vi "Dashboard Main.vi"() -> ()   [LabVIEW 2019]
uses:
  <vilib>/Rock Robotics/Network Tables/NT Read Numeric Array.vi
  <vilib>/Rock Robotics/Network Tables/NT Read Boolean.vi
  <vilib>/Rock Robotics/Network Tables/NT Read Number.vi
  <vilib>/Rock Robotics/Network Tables/NT Write Boolean.vi
  <vilib>/Rock Robotics/Network Tables/NT Write Number.vi
panel:
  out "Camera Perf":string
  in  "Camera Settings":T1={"Frame Rate"=30, "Compression"=30, "Size"=1, "DB Camera Config"=FALSE} {"Frame Rate" scale=1.0..30.0; "Compression" scale=100.0..-1.0; "Size" items=["640x480", "320x240", "160x120"]}
  in  "TCP":refnum<k5>
  out "Robot IP":string
  in  "Dashboard Tab":enum32{"Drive", "Basic", "Custom", "Variables"}(tab)
  in  "Select Auto":string(combo)="Select Autonomous ..."
  out "NT Connection":bool
  out "MotorChart R":cluster{"Numeric":dbl, "Numeric":dbl}(graph)
  out "MotorChart L":cluster{"Numeric":dbl, "Numeric":dbl}(graph)
  out "MotorSliders R":cluster{"MotorSlide1":dbl, "MotorSlide2":dbl} {"MotorSlide2" scale=-1.0..1.0 scale format="%#_2e"; "MotorSlide1" scale=-1.0..1.0 scale format="%#_2e"}
  out "MotorSliders L":cluster{"MotorSlide1":dbl, "MotorSlide2":dbl} {"MotorSlide2" scale=-1.0..1.0 scale format="%#_2e"; "MotorSlide1" scale=-1.0..1.0 scale format="%#_2e"}
  out "JS1 Z":dbl(slide) scale=-1.0..1.0 scale format="%#_2e"
  out "JS1 Graph":cluster{"X":dbl, "Y":dbl}[](graph)
  out "JS1 Buttons":T2
  out "JS2 Z":dbl(slide) scale=-1.0..1.0 scale format="%#_2e"
  out "JS2 Graph":cluster{"X":dbl, "Y":dbl}[](graph)
  out "JS2 Buttons":T2
  out "Mode":T3(ring)=enum."Auto Disabled"
  out "Background":bool
  in  "DB/String 9":string
  in  "DB/String 8":string
  in  "DB/String 7":string
  in  "DB/String 6":string
  in  "DB/String 5":string
  in  "DB/String 4":string
  in  "DB/String 3":string
  in  "DB/String 2":string
  in  "DB/String 1":string
  in  "DB/String 0":string
  in  "DB/Slider 0":dbl(slide) scale=0.0..5.0
  in  "DB/Slider 1":dbl(slide) scale=0.0..5.0
  in  "DB/Slider 2":dbl(slide) scale=0.0..5.0
  in  "DB/Slider 3":dbl(slide) scale=0.0..5.0
  out "DB/LED 3":bool
  out "DB/LED 2":bool
  out "DB/LED 1":bool
  out "DB/LED 0":bool
  in  "DB/Button 3":bool
  in  "DB/Button 2":bool
  in  "DB/Button 1":bool
  in  "DB/Button 0":bool caption="New Name"
  out "Empty":bool
  out "Full":bool
  in  "BallReset":dbl
  out "Ballons":dbl
  in  "Reset Bac":bool
  out "Encodeur":dbl
  in  "Control":dbl(slide) scale=-1.0..1.0
  out "Crochet":bool
  out "Descendue":bool
  out "Active":bool
  out "nombre tour/min":dbl
  out "on 4":bool
  out "couleur acomplis":bool
  out "?":bool
  out "on":bool
  out "decendue":bool
  out "Tree":string(tree)
  out "Camera Image":T4(plugin-control)
  in  "Camera Name":string(combo)="No Camera Selection"
  # "HW"
  # "Joysticks"
  # "Drive Motors"
  # "Front"
  # "Right"
  # "Left"
  # "Back"
  # "Elevateur"
  # "balailleuse"
  # "lanceur"
  # "tourne-disque"
  # "tour acomplis"
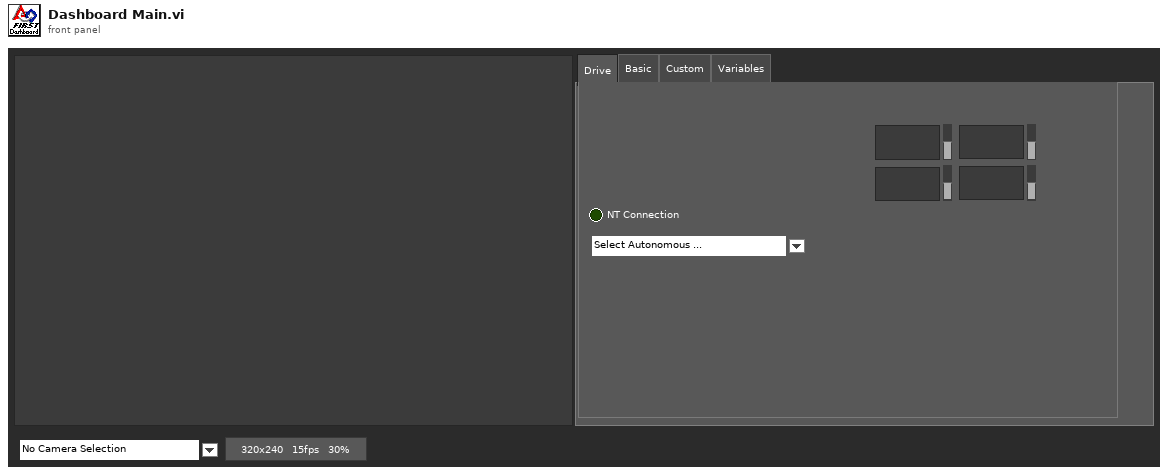
[diagram p1: front panel]
types:
  T1 = cluster{"Frame Rate":i32, "Compression":i32, "Size":u16, "DB Camera Config":bool}
  T2 = cluster{bool, bool, bool, bool, bool, bool, bool, bool, bool, bool, bool, bool}
  T3 = enum8{"Tele-Op Disabled", "Tele-Op Enabled", "Auto Disabled", "Auto Enabled", "Test Disabled", "Test Enabled", "Disconnected", "No Code", "E-Stop"}
  T4 = typedef "IMAQ Image.ctl" = refnum<image>
  T5 = cluster{"Save Path":path, "Interval (s)":dbl, "Keep":i32}
  T6 = typedef "Image Type" = u32
  T7 = cluster{"Camera Image":refnum<vi>, "Dashboard Tab":refnum<vi>, "Background":refnum<vi>, "Tree":refnum<vi>, "Camera Settings":refnum<vi>, "Camera Name":refnum<vi>, "Camera Perf":refnum<vi>}
  T8 = cluster{"Shift":bool, "Ctrl":bool, "Alt":bool, "Cmd":bool, "Opt":bool}
  T9 = cluster{"Error Strings":string, "Disable Counts":cluster{u16, u16}, "Rail Faults":cluster{u16, u16, u16}, "Robot IP":string, "DB Mode":u8, "Event Info":cluster{"Name":string, "Type":u8, "Number":u16, "Replay":u8}}
  T10 = cluster{"Storage":cluster{"Disk Free":u64, "RAM Block":u32, "RAM free":u32}, "CPU Utilization":cluster{"CPU % ISR":sgl, "CPU % Time Crit":sgl, "CPU % Timed Str":sgl, "CPU % High":sgl, "CPU % Above":sgl, "CPU % Normal":sgl, "CPU % Low":sgl}, "CAN":cluster{"% Bus Utilization":sgl, "Bus Off Cnt":u32, "TX_FIFO Full Cnt":u32, "Receive Error Cnt":u8, "Transmit Error Cnt":u8}, "HID":cluster{"HID Outputs":u32, "Rumble Low":u16, "Rumble High":u16}[]}
  T11 = cluster{"Status bits":cluster{"Test Mode":bool, "Autonomous":bool, "Enabled":bool, "Code Start":bool, "Brownout":bool, "Reserved 2":bool, "Reserved 3":bool, "E-Stop":bool}, "Code Trace":cluster{"Disabled":bool, "TeleOp":bool, "Auto":bool, "Test":bool}, "Controller Type":enum16{"unknown", "cRIO", "roboRio"}, "Code?":enum16{"unknown", "noCode", "code"}, "Battery V":dbl}
  T12 = cluster{"Control Bits":cluster{"TestMode":bool, "Autonomous":bool, "Enabled":bool, "FMS Present":bool, bool, bool, bool, "E-Stop":bool}, "Team Station ":u8, "Countdown":sgl, "Joystick Values":cluster{"Axes":dbl[], "Buttons":bool[], "POVs":i16[]}[]}
  T13 = cluster{"Axes":dbl[], "Buttons":bool[], "POVs":i16[]}[]
  T14 = cluster{"Axes":dbl[], "Buttons":bool[], "POVs":i16[]}
  T15 = cluster{"Buttons[0]":bool, "Buttons[1]":bool, "Buttons[2]":bool, "Buttons[3]":bool, "Buttons[4]":bool, "Buttons[5]":bool, "Buttons[6]":bool, "Buttons[7]":bool, "Buttons[8]":bool, "Buttons[9]":bool, "Buttons[10]":bool, "Buttons[11]":bool}
  T16 = cluster{"Camera Name":string, "Camera File Name":string, "Saved DB Images Info":cluster{"Save Path":path, "Interval (s)":dbl, "Keep":i32}}
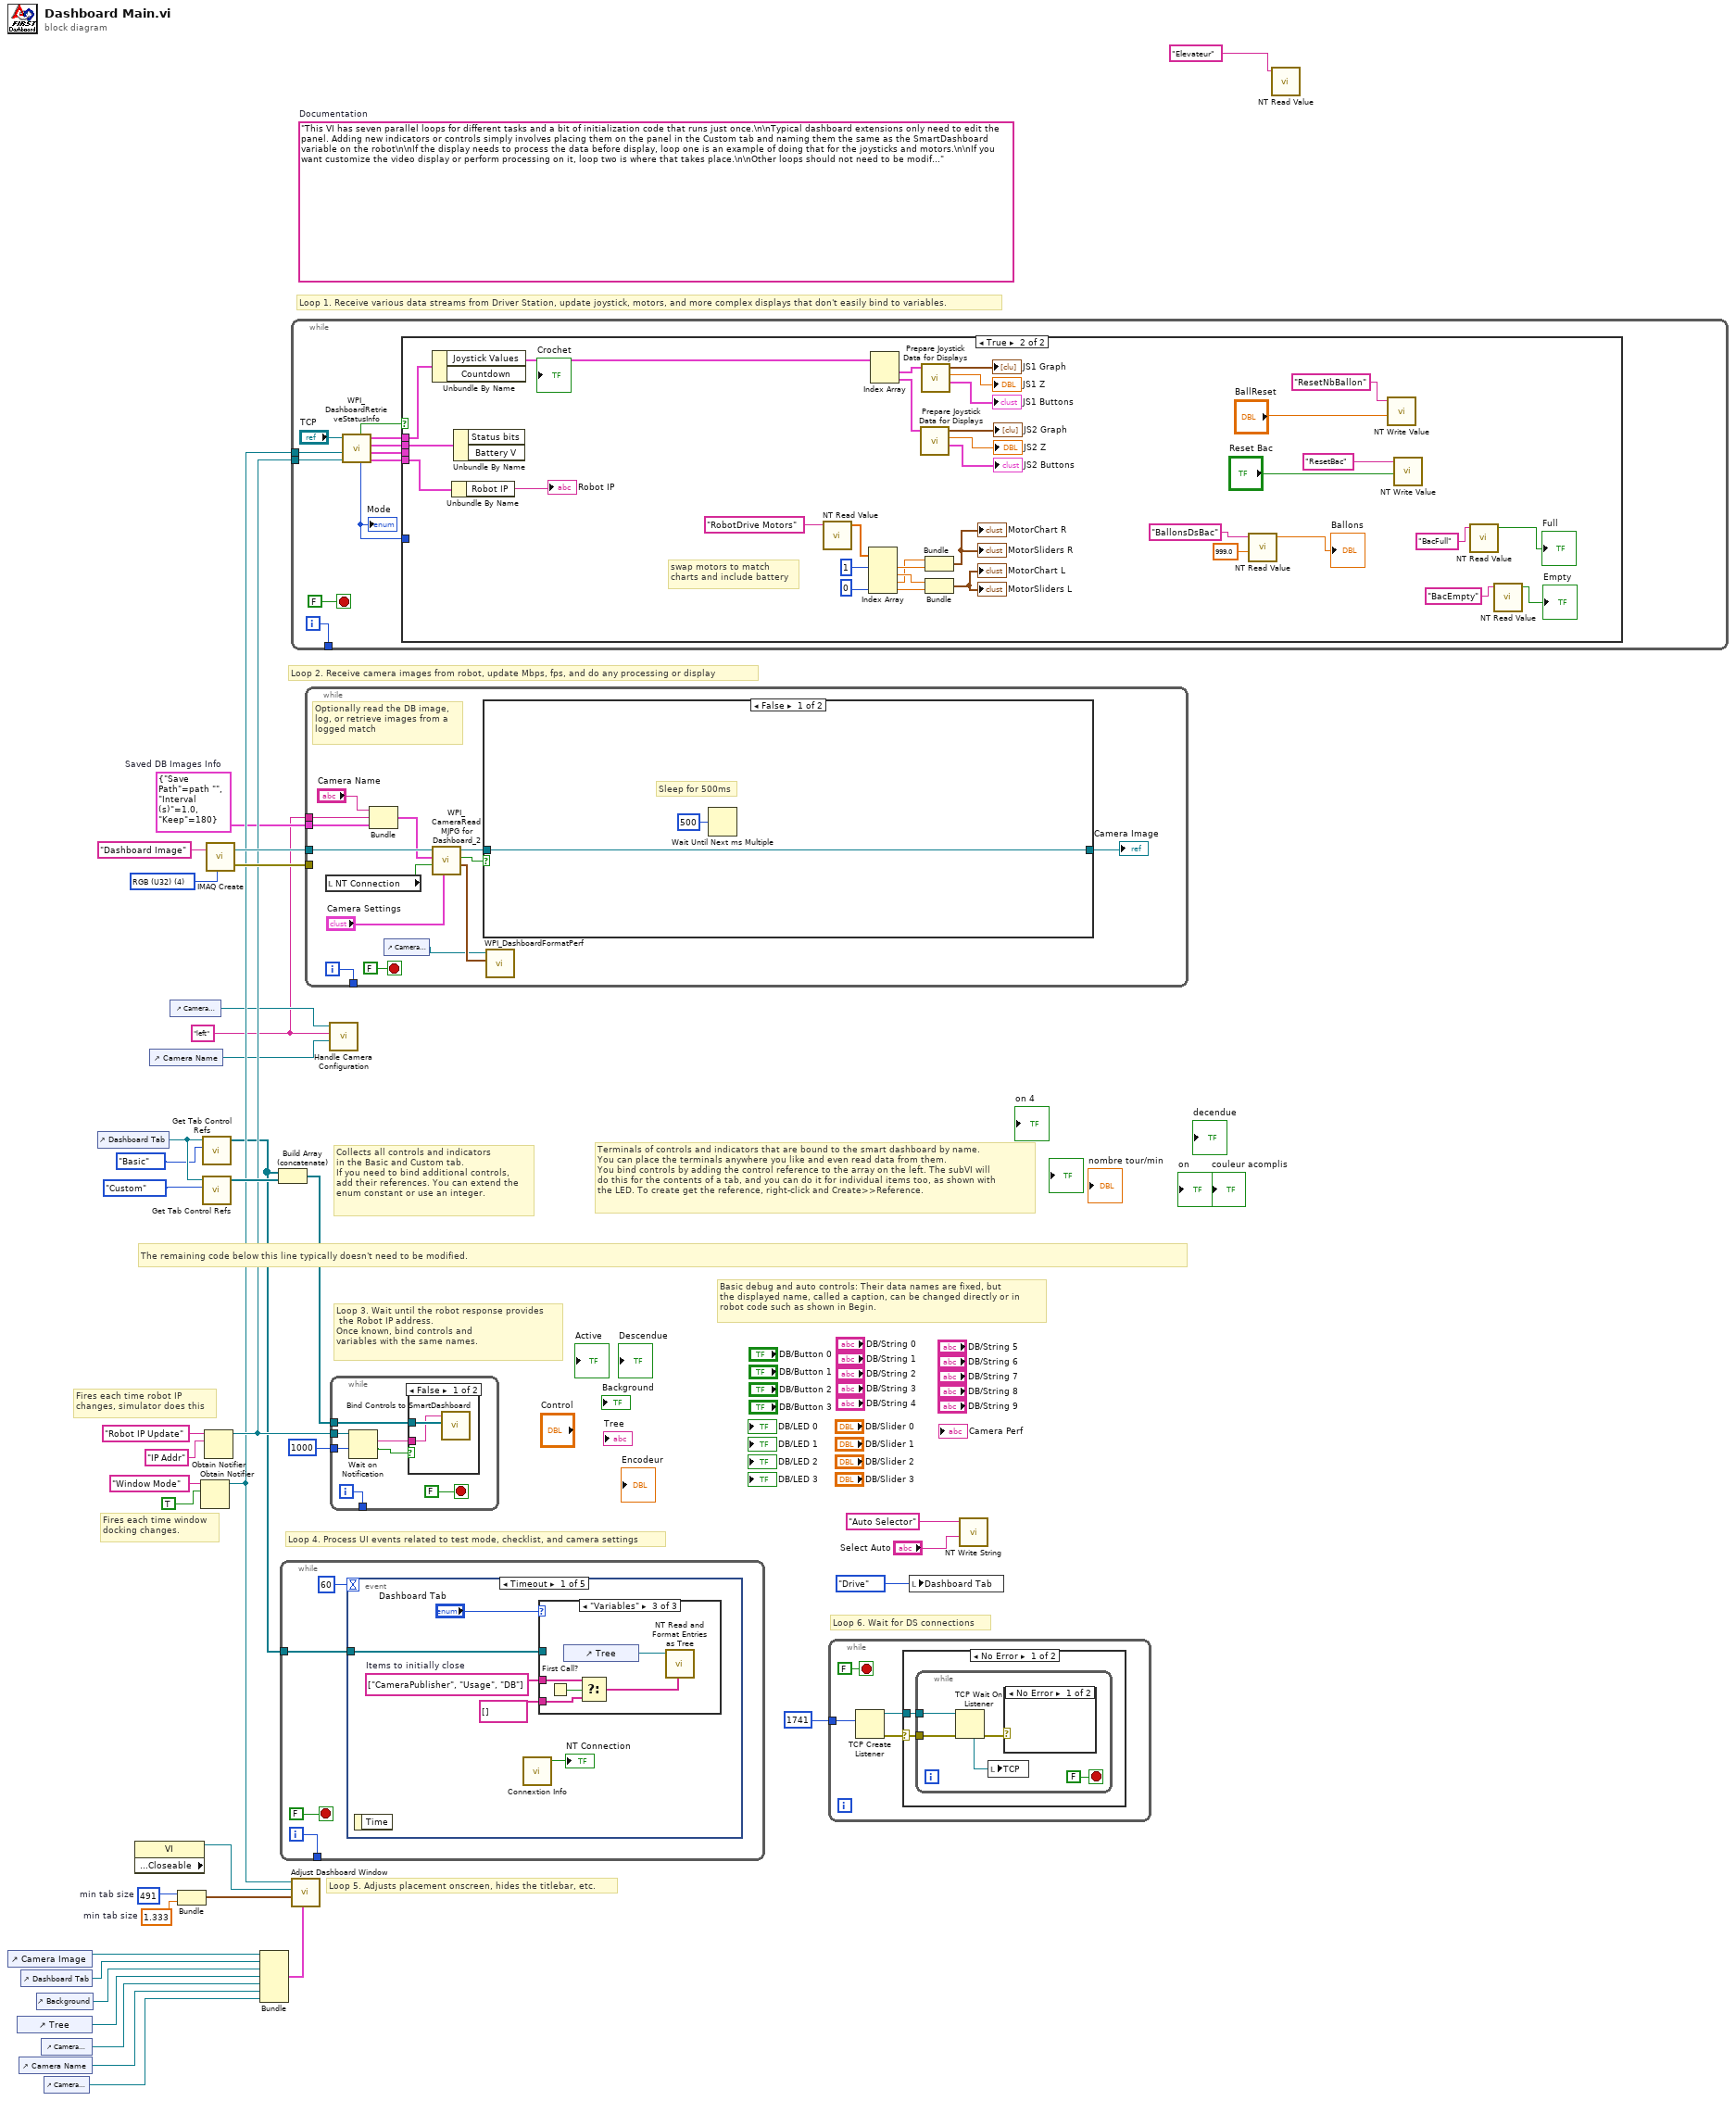
[diagram p0: block diagram]
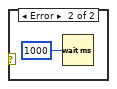
[diagram p2: hidden frame]
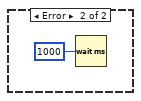
[diagram p3: hidden frame]
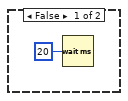
[diagram p4: hidden frame]
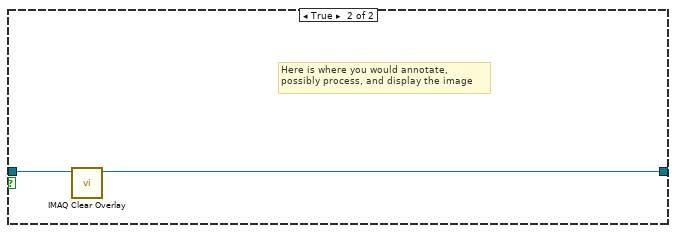
[diagram p6: hidden frame]
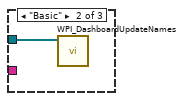
[diagram p8: hidden frame]
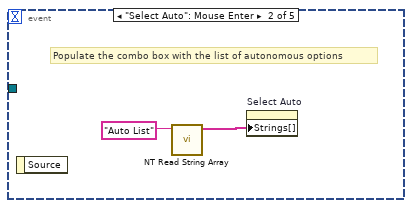
[diagram p9: hidden frame]
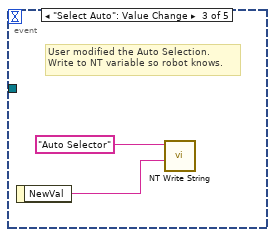
[diagram p10: hidden frame]
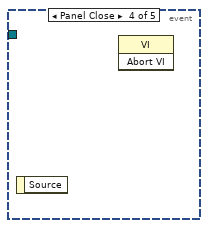
[diagram p11: hidden frame]
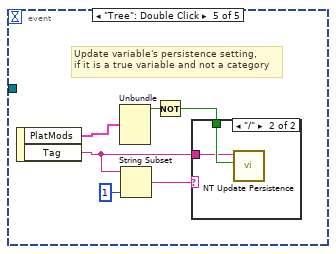
[diagram p12: hidden frame]
diagram:
  w2 = "left" ("Camera File Name")
  w3 = T5 {"Save Path"=path "", "Interval (s)"=1.0, "Keep"=180}  # Saved DB Images Info
  w23 = 491  # min tab size
  w22 = 1.333  # min tab size
  (unwired) "This VI has seven parallel loops for different tasks and a bit of initialization code that runs just once.\n\nTypical dashboard extensions only need to edit the panel. Adding new indicators or controls simply involves placing them on the panel in the Custom tab and naming them the same as the SmartDashboard variable on the robot\n\nIf the display needs to process the data before display, loop one is an example of doing that for the joysticks and motors.\n\nIf you want customize the video display or perform processing on it, loop two is where that takes place.\n\nOther loops should not need to be modified. They are pretty standard, and document the task they perform."  # Documentation
  w38 = T6 4 items=["Grayscale (U8)", "Grayscale (I16)", "Grayscale (SGL)", "Complex (CSG)", "RGB (U32)", "HSL (U32)", "RGB (U64)"] ("Image Type")
  # "Loop 6. Wait for DS connections"
  # "Basic debug and auto controls: Their data names are fixed, but\nthe displayed name, called a caption, can be changed directly or in\nrobot code such as shown in Begin."
  # "Fires each time robot IP\nchanges, simulator does this"
  # "Fires each time window\ndocking changes."
  # "Collects all controls and indicators\nin the Basic and Custom tab.\nIf you need to bind additional controls,\nadd their references. You can extend the\nenum constant or use an integer."
  # "The remaining code below this line typically doesn't need to be modified."
  # "Loop 4. Process UI events related to test mode, checklist, and camera settings"
  # "Terminals of controls and indicators that are bound to the smart dashboard by name.\nYou can place the terminals anywhere you like and even read data from them.\nYou bind controls by adding the control reference to the array on the left. The subVI will\ndo this for the contents of a tab, and you can do it for individual items too, as shown with\nthe LED. To create get the reference, right-click and Create>>Reference."
  # "Loop 3. Wait until the robot response provides\n the Robot IP address.\nOnce known, bind controls and\nvariables with the same names."
  # "Loop 5. Adjusts placement onscreen, hides the titlebar, etc."
  # "Loop 1. Receive various data streams from Driver Station, update joystick, motors, and more complex displays that don't easily bind to variables."
  # "Loop 2. Receive camera images from robot, update Mbps, fps, and do any processing or display"
  n1 = control-ref of="Camera Image"() -> (w25:refnum<vi>)
  n2 = control-ref of="Tree"() -> (w9:refnum<vi>)
  n3 = control-ref of="Camera Name"() -> (w7:refnum<vi>)
  n4 = control-ref of="Dashboard Tab"() -> (w24:refnum<vi>)
  n5 = control-ref of="Background"() -> (w20:refnum<vi>)
  n6 = control-ref of="Camera Settings"() -> (w8:refnum<vi>)
  n7 = control-ref of="Camera Perf"() -> (w6:refnum<vi>)
  n8 = control-ref of="Dashboard Tab"() -> (w28:refnum<vi>)
  n9 = property class="VI" props=["Front Panel.Closeable"]() -> (reference out=w29:refnum<vi>)  [unwired: 2 in, 2 out]
  n10 = control-ref of="Camera Name"() -> (w13:refnum<vi>)
  n11 = control-ref of="Camera Settings"() -> (w14:refnum<vi>)
  n12 = Bundle("min tab size"=w23, "min tab size"=w22) -> (w21:cluster{"min tab size":i32, "min tab size":dbl})  [unwired: 1 in]
  n13 = Obtain Notifier(name (unnamed)="Window Mode", notification data type=TRUE) -> (notifier out=w17:refnum<notifier>)  [unwired: 2 in, 2 out]
  n14 = call <vilib>:"Get Tab Control Refs.vi"("Page Index"=enum32{"Drive", "Basic", "Custom", "Variables"}."Basic" ("Dashboard Tab"), "TabControl in"=w28) -> ("ControlsOnPage"=w12:refnum<vi>[])  [unwired: 9 in]
  n15 = call <vilib>:"Get Tab Control Refs.vi"("Page Index"=enum32{"Drive", "Basic", "Custom", "Variables"}."Custom" ("Dashboard Tab"), "TabControl in"=w28) -> ("ControlsOnPage"=w27:refnum<vi>[])  [unwired: 9 in]
  n16 = Obtain Notifier(name (unnamed)="Robot IP Update", notification data type="IP Addr" ("name (unnamed)")) -> (notifier out=w18:refnum<notifier>)  [unwired: 2 in, 2 out]
  n17 = call "IMAQ Create"("Image Name"="Dashboard Image", "Image Type"=w38) -> ("New Image"=w36:T4, "error out"=w35:errorcluster)  [unwired: 2 in, 1 out]
  n18 = Bundle("Camera Image"=w25, "Dashboard Tab"=w24, "Background"=w20, "Tree"=w9, "Camera Settings"=w8, "Camera Name"=w7, "Camera Perf"=w6) -> (w19:T7)  [unwired: 1 in]
  n19 = Build Array (concatenate)(w12, w27) -> (w26:refnum<vi>[])
  n20 = while {
    tunnel: [w40] -> _
    tunnel: w12 -> [w39]
    i -> [w40]
    stop <- FALSE stop-if-true
    n21 = event shown="[0] Timeout" {
      selector: _ -> [_ _ _ _ _]
      dyn-events: _ -> [_ _ _ _ _]
      timeout: u32 60 ("milliseconds to wait") -> [_ _ _ _ _]
      tunnel: w39 -> [w45 _ _ _ _]
      event Timeout {
        w44 = string[] ["CameraPublisher", "Usage", "DB"]  # Items to initially close
        n22 = event-data() -> ()  [unwired: 1 in, 1 out]
        n23 = call <vilib>:"Connextion Info.vi"() -> ("Connected"=→"NT Connection":bool)  [unwired: 10 in, 1 out]
        n24 = case shown="\"Variables\"" "Dashboard Tab" {
          tunnel: w45 -> [_ w48 _]
          tunnel: w44 -> [_ _ w51]
          tunnel: string[] [] -> [_ _ w50]
          frame "Custom", Default {
          }
          frame "Basic" {
            n25 = call <vilib>:"WPI_DashboardUpdateNames.vi"("Controls on Tab"=w48) -> ()  [unwired: 11 in]
          }
          frame "Variables" {
            n26 = First Call?() -> (First Call?: T/F=w52:bool)
            n27 = control-ref of="Tree"() -> (w53:refnum<vi>)
            n28 = Select(t=w51, s=w52, f=w50) -> (s? t:f=w49:string[])
            n29 = call <vilib>:"NT Read and Format Entries as Tree.vi"("Tags to  Close"=w49, "Tree Refnum"=w53) -> ()  [unwired: 8 in, 2 out]
          }
        }
      }
      event "Select Auto": Mouse Enter {
        # "Populate the combo box with the list of autonomous options"
        n30 = event-data() -> ()  [unwired: 1 in, 1 out]
        n31 = call <vilib>:"NT Read String Array.vi"("Name"="Auto List") -> ("String Array"=w54:string[])  [unwired: 9 in, 1 out]
        n32 = property on="Select Auto" class="CmbBox"("Strings[]"=w54) -> ()  [unwired: 2 in, 2 out]
      }
      event "Select Auto": Value Change {
        # "User modified the Auto Selection.\nWrite to NT variable so robot knows."
        n33 = event-data() -> ("NewVal"=w56:string)  [unwired: 1 in]
        n34 = call <vilib>:"NT Write String.vi"("String"=w56, "Name"="Auto Selector") -> ()  [unwired: 9 in, 1 out]
      }
      event Panel Close {
        n35 = event-data() -> ()  [unwired: 1 in, 1 out]
        n36 = invoke class="VI" method="Abort VI"() -> ()  [unwired: 3 in, 3 out]
      }
      event "Tree": Double Click {
        # "Update variable's persistence setting,\nif it is a true variable and not a category"
        n37 = event-data() -> ("PlatMods"=w59:T8, "Tag"=w58:string)  [unwired: 1 in]
        n38 = Unbundle(w59) -> ("Shift"=w63:bool)  [unwired: 4 out]
        n39 = String Subset(string=w58, length (rest)=1 ("length (rest)")) -> (substring=w60:string)  [unwired: 1 in]
        n40 = Not(x=w63) -> (.not. x?=w62:bool)
        n41 = case shown="\"/\"" w60 {
          tunnel: w62 -> [_ w65]
          tunnel: w58 -> [_ w64]
          frame Default {
          }
          frame "/" {
            n42 = call <vilib>:"NT Update Persistence.vi"("Persistence"=w65, "Name"=w64) -> ()  [unwired: 9 in, 1 out]
          }
        }
      }
    }
  }
  n43 = while {
    tunnel: [w75] -> _
    tunnel: w18 -> [w69]
    tunnel: w17 -> [w66]
    i -> [w75]
    stop <- FALSE stop-if-true
    n44 = call <vilib>:"WPI_DashboardRetrieveStatusInfo.vi"("Binding Refnum"=w69, "Window Mode Notifier"=w66, "TCP Cnx"="TCP") -> ("Power and Errors"=w70:T9, "Robot Metrics"=w73:T10, "Status Info"=w74:T11, "Control Info"=w71:T12, "Robot Mode"=w68:T3, "Process?"=w72:bool)  [unwired: 3 in]
    "Mode" <- w68
    n45 = case shown="True" w72 {
      tunnel: w74 -> [_ w111]
      tunnel: w73 -> [_ _]
      tunnel: w71 -> [_ w110]
      tunnel: w70 -> [_ w109]
      tunnel: w68 -> [_ _]
      frame False {
        n46 = Wait (ms)(milliseconds to wait=u32 20) -> ()  [unwired: 1 out]
      }
      frame True {
        # "swap motors to match\ncharts and include battery"
        n47 = Unbundle By Name(w110) -> ("Joystick Values"=w100:T13)  [unwired: 1 out]
        n48 = Unbundle By Name(w109) -> ("Robot IP"=→"Robot IP":string)
        n49 = Unbundle By Name(w111) -> ()  [unwired: 2 out]
        n50 = call-poly <vilib>:"NT Read Value.vi"("Name"="RobotDrive Motors") -> ("Numeric Array"=w90:dbl[])  [unwired: 9 in, 1 out]
        n51 = Index Array(array=w90, index #1=1, index #4=0) -> (element #1=w104:dbl, element #2=w105:dbl, element #3=w103:dbl, element #4=w108:dbl)  [unwired: 2 in]
        n52 = Index Array(array=w100) -> (element #1=w99:T14, element #2=w95:T14)  [unwired: 2 in]
        n53 = call "Prepare Joystick Data for Displays.vi"("Joystick Values"=w95) -> ("Buttons"=→"JS2 Buttons":T15, "Z Axis"=→"JS2 Z":dbl, "Cartesian Data"=→"JS2 Graph":cluster{"X axis":dbl, "X axis":dbl}[])  [unwired: 8 in]
        n54 = call "Prepare Joystick Data for Displays.vi"("Joystick Values"=w99) -> ("Buttons"=→"JS1 Buttons":T15, "Z Axis"=→"JS1 Z":dbl, "Cartesian Data"=→"JS1 Graph":cluster{"X axis":dbl, "X axis":dbl}[])  [unwired: 8 in]
        n55 = Bundle("Numeric"=w103, "Numeric"=w104) -> (→"MotorChart R" →"MotorSliders R":cluster{"Numeric":dbl, "Numeric":dbl})  [unwired: 1 in]
        n56 = Bundle("Numeric"=w105, "Numeric"=w108) -> (→"MotorChart L" →"MotorSliders L":cluster{"Numeric":dbl, "Numeric":dbl})  [unwired: 1 in]
        n57 = call-poly <vilib>:"NT Read Value.vi"("Default Value"=999.0, "Name"="BallonsDsBac") -> ("Numeric"=→"Ballons":dbl)  [unwired: 8 in, 1 out]
        n58 = call-poly <vilib>:"NT Write Value.vi"("Numeric"="BallReset", "Name"="ResetNbBallon") -> ()  [unwired: 9 in, 1 out]
        n59 = call-poly <vilib>:"NT Write Value.vi"("Boolean"="Reset Bac", "Name"="ResetBac") -> ()  [unwired: 9 in, 1 out]
        n60 = call-poly <vilib>:"NT Read Value.vi"("Name"="BacFull") -> ("Boolean"=→"Full":bool)  [unwired: 9 in, 1 out]
        n61 = call-poly <vilib>:"NT Read Value.vi"("Name"="BacEmpty") -> ("Boolean"=→"Empty":bool)  [unwired: 9 in, 1 out]
      }
    }
  }
  n62 = call "Adjust Dashboard Window.vi"("Sizing Refnums"=w19, "Size Constraints"=w21, "VI"=w29, "WIn Mode"=w17) -> ()  [unwired: 8 in]
  n63 = while {
    tunnel: w36 -> [w123]
    tunnel: w35 -> [_]
    tunnel: [w124] -> _
    tunnel: w3 -> [w117]
    tunnel: w2 -> [w114]
    i -> [w124]
    stop <- FALSE stop-if-true
    # "Optionally read the DB image,\nlog, or retrieve images from a\nlogged match"
    n64 = local read "NT Connection"() -> (w118:bool)
    n65 = Bundle("Camera Name"="Camera Name", "Camera File Name"=w114, "Saved DB Images Info"=w117) -> (w116:T16)  [unwired: 1 in]
    n66 = control-ref of="Camera Perf"() -> (w112:refnum<vi>)
    n67 = call <vilib>:"WPI_CameraRead MJPG for Dashboard_2.vi"("Camera Settings"="Camera Settings", "NT Connection"=w118, "Capture Info"=w116, "Image in"=w123) -> ("perf info"=w113:cluster{"Bandwidth (Mbps)":dbl, "fps":dbl}, "Active"=w121:bool, "Image\\ out"=w122:T4)  [unwired: 5 in]
    n68 = case shown="False" w121 {
      tunnel: w122 -> [w126 w129]
      tunnel: [w126 w128] -> w119
      frame False {
        # "Sleep for 500ms"
        n69 = Wait Until Next ms Multiple(millisecond multiple=u32 500) -> ()  [unwired: 1 out]
      }
      frame True {
        # "Here is where you would annotate,\npossibly process, and display the image"
        n70 = call "IMAQ Clear Overlay"("Image"=w129) -> ("Image Out"=w128:T4)  [unwired: 2 in, 8 out]
      }
    }
    "Camera Image" <- w119
    n71 = call <vilib>:"WPI_DashboardFormatPerf.vi"("Performance"=w113, "String in"=w112) -> ()  [unwired: 10 in]
  }
  n72 = call "Handle Camera Configuration.vi"("CameraNameRef"=w13, "Display Name"=w2, "ClusterRef"=w14) -> ()  [unwired: 9 in]
  n73 = while {
    tunnel: w26 -> [w136]
    tunnel: w18 -> [w134]
    tunnel: [w132] -> _
    tunnel: u32 1000 ("milliseconds to wait") -> [w131]
    i -> [w132]
    stop <- FALSE stop-if-true
    n74 = Wait on Notification(notifier=w134, timeout in ms (-1)=w131) -> (notification=w133:string, timed out?=w130:bool)  [unwired: 2 in, 2 out]
    n75 = case shown="False" w130 {
      tunnel: w136 -> [w138 _]
      tunnel: w133 -> [w137 _]
      frame False {
        n76 = call <vilib>:"Bind Controls to SmartDashboard.vi"("Bound Control Refs"=w138, "Server IP Address"=w137) -> ()  [unwired: 10 in]
      }
      frame True {
      }
    }
  }
  n77 = while {
    tunnel: u16 1741 ("timeout ms (25000)") -> [w140]
    stop <- FALSE stop-if-true
    n78 = TCP Create Listener(10:w140) -> (0:w139:errorcluster, 3:w141:refnum<k5>)  [unwired: 4 in, 1 out]
    n79 = case shown="No Error" w139 {
      selector: w139 -> [w143 _]
      tunnel: w141 -> [w144 _]
      frame No Error {
        n80 = while {
          tunnel: w144 -> [w147]
          tunnel: w143 -> [w146]
          stop <- FALSE stop-if-true
          n81 = TCP Wait On Listener(8:w146, 11:w147) -> (0:w148:errorcluster, 4:w149:refnum<k5>)  [unwired: 2 in, 3 out]
          n82 = local write "TCP"(w149) -> ()
          n83 = case shown="No Error" w148 {
            frame No Error {
            }
            frame Error {
              n84 = Wait (ms)(milliseconds to wait=u32 1000) -> ()  [unwired: 1 out]
            }
          }
        }
      }
      frame Error {
        n85 = Wait (ms)(milliseconds to wait=u32 1000) -> ()  [unwired: 1 out]
      }
    }
  }
  n86 = local write "Dashboard Tab"(enum32{"Drive", "Basic", "Custom", "Variables"}."Drive" ("Dashboard Tab")) -> ()
  n87 = call <vilib>:"NT Write String.vi"("String"="Select Auto", "Name"="Auto Selector") -> ()  [unwired: 9 in, 1 out]
  n88 = call-poly <vilib>:"NT Read Value.vi"("Name"="Elevateur" ("refnum name")) -> ()  [unwired: 9 in, 2 out]
